vi "PH_PPMA_PowerUnit.ProcPeriodic.vi"(0 "i ref in":refnum<vi>, 3 "ms timeout (100)":i32=100, 5 "error in (no error)":errorcluster) -> (14 "i ref out":refnum<vi>, 17 "timed out":bool, 19 "error out":errorcluster)   [LabVIEW 2014, in "PH_PPMA_PowerUnit.lvlib"]
doc: "This method serves to periodically do things like reading values from the HW. Methods that should be executed periodically should be called from THIS methode. Add code here."
uses:
  PH_PPMA_PowerUnit.lvlib
  CSCore/CSSystem/CSSystemLib/CSSystemLib.lvlib
  CSCore/BaseProcess/BaseProcess.lvlib
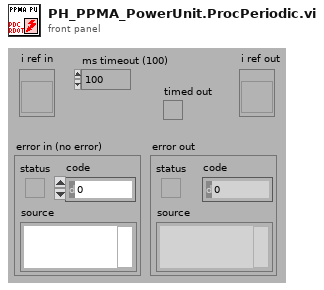
[diagram p1: front panel]
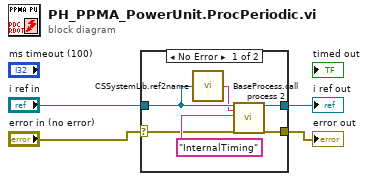
[diagram p0: block diagram]
diagram:
  n1 = case shown="No Error" "error in (no error)" {
    selector: "error in (no error)" -> [w5 w11]
    tunnel: [w9 w12] -> w4
    tunnel: [w8 w11] -> w3
    tunnel: "i ref in" -> [w7 w12]
    frame No Error {
      n2 = call "CSSystemLib.ref2name.vi"("obj refnum"=w7) -> ("name"=w6:string)
      n3 = call "BaseProcess.call process 2.vi"("i ref in"=w7, "Object"=w6, "Selector"="InternalTiming", "error in (no error)"=w5) -> ("i ref out"=w9:refnum<vi>, "error out"=w8:errorcluster)  [unwired: 14 in]
    }
    frame Error {
    }
  }
  "error out" <- w3
  "i ref out" <- w4
